vi "Read Configuration.vi"(8 "error in (no error)":errorcluster, 11 "Status 2":T1) -> (0 "error out":errorcluster, 3 "Status":T1)   [LabVIEW 2016]
doc: "This VI will read in the client configuration and provide the default configuration if the client configuration is not found"
uses:
  Controls/Database Status.ctl
  Architecture/Message Queue/Message Cluster.ctl
  Car Wash Controller/Controls/Steps.ctl
  Car Wash Controller/Controls/Stations.ctl
  Architecture/Modules.ctl
  Architecture/Message Queue/Message Queue.lvlib
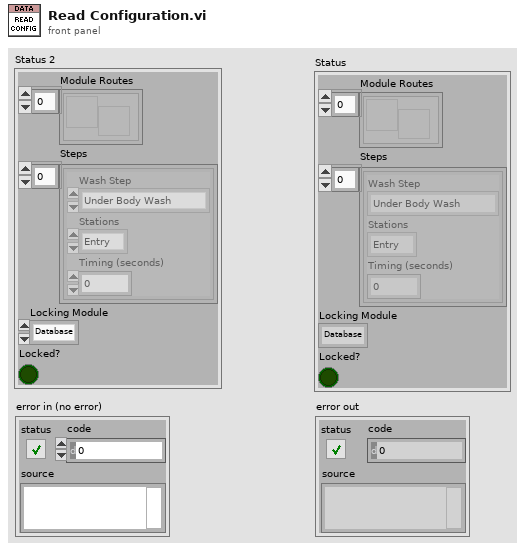
[diagram p1: front panel]
types:
  T1 = typedef "Database Status.ctl" = cluster{"Module Routes":refnum<user-event>[], "Steps":cluster{"Wash Step":T2, "Stations":T3, "Timing (seconds)":u32}[], "Locking Module":T4, "Locked?":bool}
  T2 = typedef "Steps.ctl" = enum16{"Under Body Wash", "Bug Remover", "Pre-Soak", "High Pressure Wash", "Low Pressure Wax", "Spot Free Rinse", "Tire Shine Foam", "Air Dry"}
  T3 = typedef "Stations.ctl" = enum16{"Entry", "Station 1", "Station 2", "Station 3", "Exit"}
  T4 = typedef "Modules.ctl" = enum16{"Database", "Car Wash Controller", "Console"}
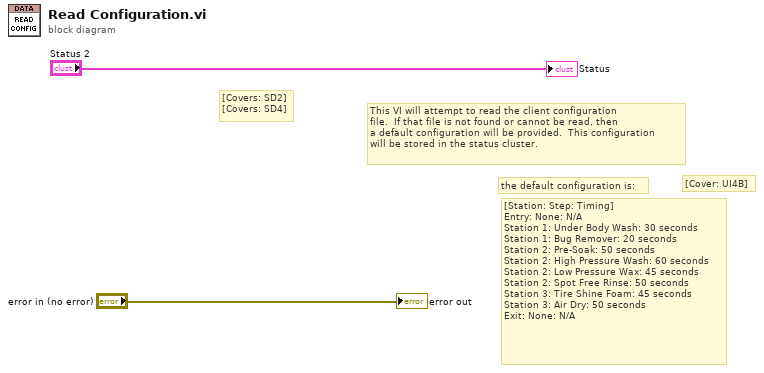
[diagram p0: block diagram]
diagram:
  # "[Cover: UI4B]"
  # "[Station: Step: Timing]\nEntry: None: N/A\nStation 1: Under Body Wash: 30 seconds\nStation 1: Bug Remover: 20 seconds\nStation 2: Pre-Soak: 50 seconds\nStation 2: High Pressure Wash: 60 seconds\nStation 2: Low Pressure Wax: 45 seconds\nStation 2: Spot Free Rinse: 50 seconds\nStation 3: Tire Shine Foam: 45 seconds\nStation 3: Air Dry: 50 seconds\nExit: None: N/A"
  # "the default configuration is:"
  # "This VI will attempt to read the client configuration\nfile.  If that file is not found or cannot be read, then\na default configuration will be provided.  This configuration\nwill be stored in the status cluster."
  # "[Covers: SD2]\n[Covers: SD4]"
  "error out" <- "error in (no error)"
  "Status" <- "Status 2"
